vi "PI_E709_start.vi"() -> ()   [LabVIEW 2012]
panel:
  out "Identification":string
  in  "Position values":dbl[](array[numeric]) format="%.6f"
  out "Position":dbl[](array[numeric]) format="%.6f"
  out "Stage names":string[](array[string])
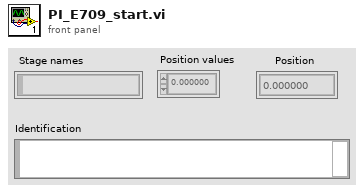
[diagram p1: front panel]
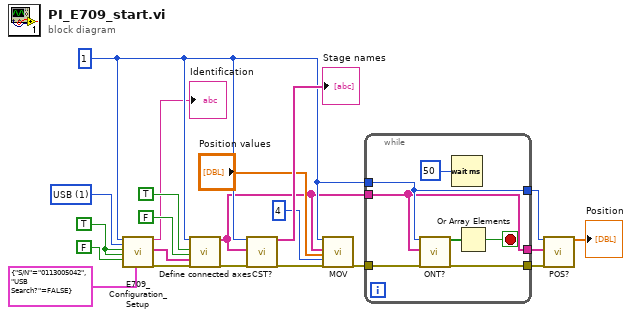
[diagram p0: block diagram]
diagram:
  w13 = TRUE ("Connected?")
  w21 = u16 1 items=["RS232", "USB"] ("Interface")
  w11 = 1 ("System no.")
  n1 = call "E709_Configuration_Setup.vi"("System no."=w11, "Interface"=w21, "Connected?"=w13, "Change servo status to ON?"=w13, "Perform autozero?"=FALSE, "USB settings"=cluster{"S/N":string, "USB Search?":bool} {"S/N"="0113005042", "USB Search?"=FALSE}) -> ("Identification"=→"Identification":string, "Conn. \nAxis"=w19:string[], "error out"=w9:errorcluster)  [unwired: 8 in, 3 out]
  n2 = call "Define connected axes.vi"("System no."=w11, "Read from\ncontroller?"=TRUE ("Read from\ncontroller?"), "Invert\norder?"=FALSE ("Invert\norder?"), "Conn. axes"=w19, "error in"=w9) -> ("Conn. Axes out"=w10:string[], "error out"=w8:errorcluster)  [unwired: 13 in]
  n3 = call "CST?.vi"("System no."=w11, "Axes to query"=w10, "error in"=w8) -> ("Stage names"=→"Stage names":string[], "error out"=w2:errorcluster)  [unwired: 15 in]
  n4 = call "MOV.vi"("System no."=w11, "Axes to move"=w10, "Position values"="Position values", "No.of digits"=i16 4, "error in"=w2) -> ("error out"=w7:errorcluster)  [unwired: 14 in]
  n5 = while {
    tunnel: w11 -> [w26]
    tunnel: w10 -> [w25]
    tunnel: w7 -> [w28]
    tunnel: [w27] -> w6
    tunnel: [w26] -> w4
    tunnel: [w25] -> w3
    stop <- w23 stop-if-true
    n6 = call "ONT?.vi"("System no."=w26, "Axes to query"=w25, "error in"=w28) -> ("Axis on target?"=w24:bool[], "error out"=w27:errorcluster)  [unwired: 15 in]
    n7 = Wait (ms)(milliseconds to wait=u32 50 ("等待时间（毫秒）")) -> ()  [unwired: 1 out]
    n8 = Or Array Elements(Boolean array=w24) -> (logical OR=w23:bool)
  }
  n9 = call "POS?.vi"("System no."=w4, "Axes to query"=w3, "error in"=w6) -> ("Position"=→"Position":dbl[])  [unwired: 15 in, 1 out]
